vi "Session3_FlowControl.vi"() -> ()   [LabVIEW 2016]
panel:
  in  "milliseconds to wait":u32=200
  out "Thermometer":dbl(slide) scale=0.0..100.0
  out "Temp Value":dbl
  in  "Clear":bool
  out "Temp Chart":dbl(graph)
  in  "Sensor Simulator":dbl(slide) scale=0.0..100.0
  in  "stop":bool
  # "Session 3 – Project: Real-Time Temperature Display"
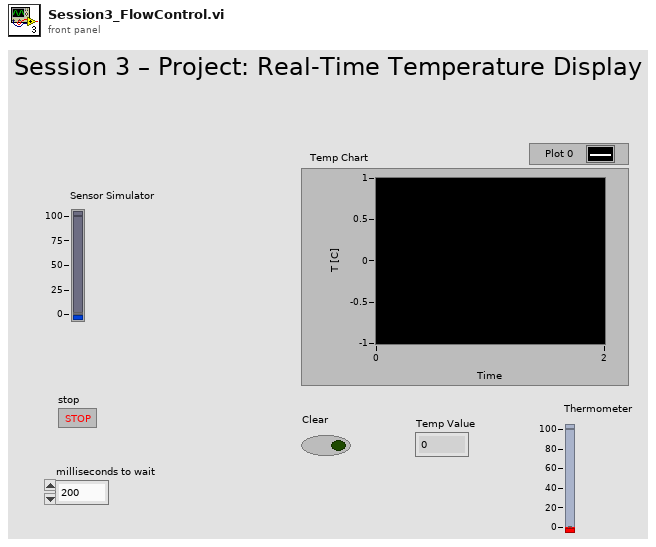
[diagram p1: front panel]
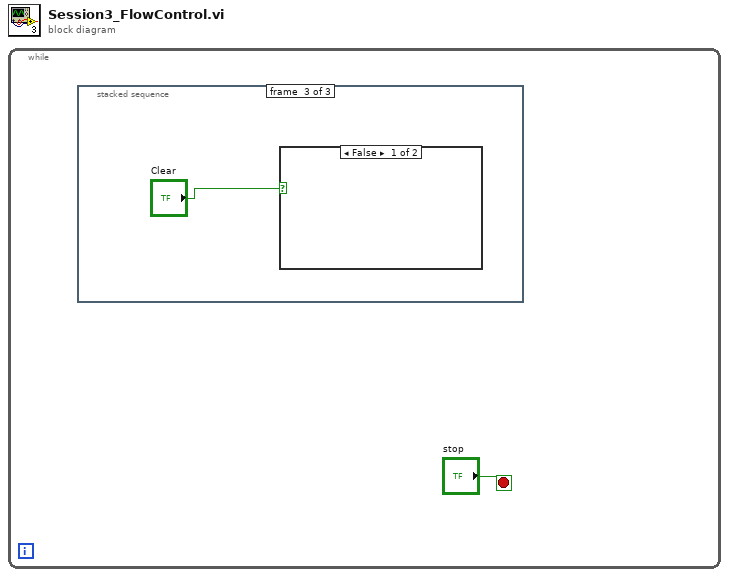
[diagram p0: block diagram]
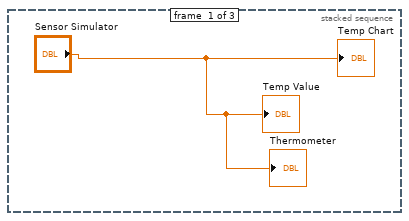
[diagram p2: hidden frame]
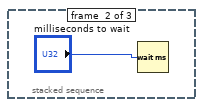
[diagram p3: hidden frame]
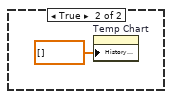
[diagram p4: hidden frame]
diagram:
  n1 = while {
    stop <- "stop" stop-if-true
    n2 = stacked-sequence {
      frame #0 {
        "Temp Chart" <- "Sensor Simulator"
        "Temp Value" <- "Sensor Simulator"
        "Thermometer" <- "Sensor Simulator"
      }
      frame #1 {
        n3 = Wait (ms)(milliseconds to wait="milliseconds to wait") -> ()  [unwired: 1 out]
      }
      frame #2 {
        n4 = case shown="False" "Clear" {
          frame False {
          }
          frame True {
            n5 = property on="Temp Chart" class="WFChart (strict)"("History Data"=dbl[] []) -> ()  [unwired: 2 in, 2 out]
          }
        }
      }
    }
  }
